vi "ReadbyWeakRefRing.vi"(8 "error in":errorcluster caption="entrée d'erreur", 11 "Control Ref":refnum<vi>) -> (0 "error out":errorcluster caption="sortie d'erreur", 3 "Valeur":u16)   [LabVIEW 2019]
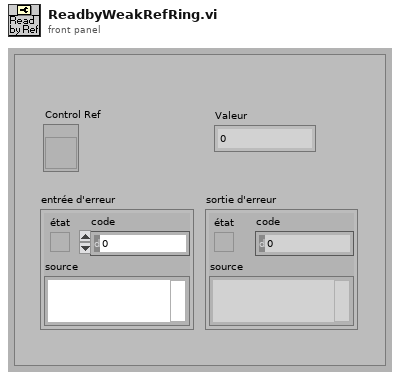
[diagram p1: front panel]
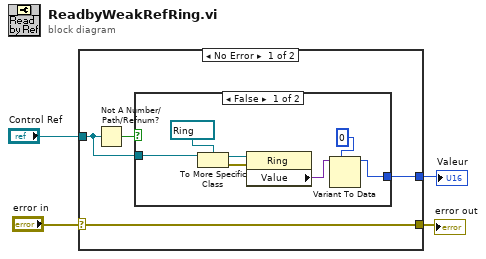
[diagram p0: block diagram]
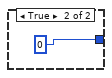
[diagram p2: hidden frame]
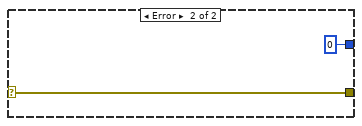
[diagram p3: hidden frame]
diagram:
  n1 = case shown="No Error" "error in" {
    selector: "error in" -> [w6 w18]
    tunnel: "Control Ref" -> [w7 _]
    tunnel: [w6 w18] -> w2
    tunnel: [w5 u16 0 ("Valeur")] -> w1
    frame No Error {
      n2 = Not A Number/Path/Refnum?(number/path/refnum=w7) -> (NaN/Path/Refnum?=w8:bool)
      n3 = case shown="False" w8 {
        tunnel: w7 -> [w12 _]
        tunnel: [w9 u8 0 ("Valeur")] -> w5
        frame False {
          n4 = To More Specific Class(target class=refnum<vi> refnum ("référence"), reference=w12) -> (specific class reference=w14:refnum<vi>, error out=w13:errorcluster)  [unwired: 1 in]
          n5 = property class="Ring"(reference=w14, error in=w13) -> ("Value"=w10:variant)  [unwired: 2 out]
          n6 = Variant To Data(type=u16 0 ("Valeur"), Variant=w10) -> (data=w9:u16)  [unwired: 1 in, 1 out]
        }
        frame True {
        }
      }
    }
    frame Error {
    }
  }
  "Valeur" <- w1
  "error out" <- w2
